vi "demod.vi"(0 "SNR":dbl, 7 "bit":bool) -> (8 "soft bit":dbl)   [LabVIEW 2017]
uses:
  <vilib>/ptbypt/NI_PtbyPt.lvlib
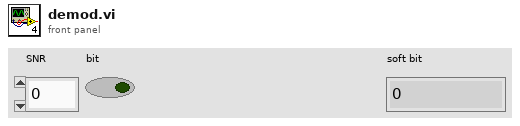
[diagram p1: front panel]
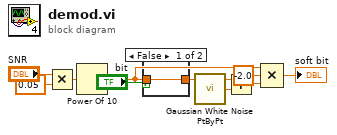
[diagram p0: block diagram]
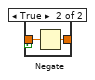
[diagram p2: hidden frame]
diagram:
  n1 = Multiply(x="SNR", y=0.05) -> (x*y=w10:dbl)
  n2 = Power Of 10(x=w10) -> (10^x=w2:dbl)
  n3 = case shown="False" "bit" {
    tunnel: w2 -> [w11 w13]
    tunnel: [w11 w12] -> w6
    frame False {
    }
    frame True {
      n4 = Negate(x=w13) -> (-x=w12:dbl)
    }
  }
  n5 = call <vilib>:"Gaussian White Noise PtByPt.vi"() -> ("Gaussian white noise"=w5:dbl)  [unwired: 3 in]
  n6 = Add(x=w6, y=w5) -> (x+y=w4:dbl)
  n7 = Compound Arithmetic op=MULTIPLY(w2, -2.0 ("y"), w4) -> (→"soft bit":dbl)
